vi "CC FITS Make FITS Header Table.vi"() -> ()   [LabVIEW 2021]
uses:
  typedefs/FITS HK Header Table.ctl
  Logging/CC enum Current Values Action.ctl
  <userlib>/gfitsio/cfitsio-bitpix.ctl
  <userlib>/gfitsio/gfitsio-write-image-subset-dbl-2d.vi
  hk-channel-class/HK Table/HK Table.lvclass
  <userlib>/gfitsio/gfitsio.lvlib
panel:
  in  "Fixed Header":bool
  in  "Test File":bool
  in  "Cancel Button":bool
  in  "OK Button":bool
  in  "Remove":bool
  in  "Add":bool
  in  "FITS Header":i32(listbox)
  in  "All Housekeeping":i32(listbox)
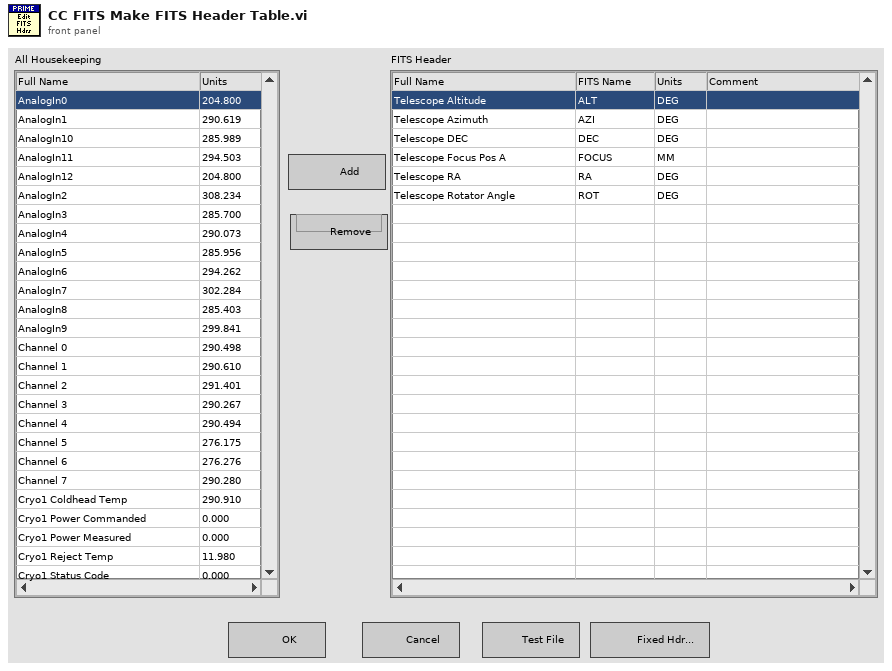
[diagram p1: front panel]
types:
  T1 = typedef "FITS HK Header Table.ctl" = cluster{"Full Name":string, "FITS Name":string, "Units":string, "Comment":string}
  T2 = cluster{"state":refnum<user-event>, "All HK":string[][], "Hdr Map":map{string, T1}, "Fixed Hdr":map{string, T1}}
  T3 = typedef "CC enum Current Values Action.ctl" = enum16{"Init", "Write Item", "Write Array", "Read Item", "Read Array", "Read All", "Add Channels", "New File", "Add Message", "Get Current Values", "Close"}
  T4 = enum16{"open", "open or create", "create", "create or replace"}
  T5 = enum16{"open", "open or create", "create or replace", "create", "open (read only)"}
  T6 = typedef "RIMAS Detector Config.ctl" = cluster{"Detector":u16, "Offsets":u16[][], "Detector Computer":T7, "FITS hdr template0":path, "FITS hdr template1":path, "FITS Data File Path":path, "FITS Detector Settings":T8, "Sim Folder":path, "Integration Mode":T9, "Integration Time":dbl, "Frame Int Time":dbl}
  T7 = typedef "RIMAS Detector Server Config.ctl" = cluster{"Machine":string, "Password":string, "FITS File Path":string, "Port":u16, "Header Path":string, "Name":string}
  T8 = typedef "RIMAS Observation Config.ctl" = cluster{"Exp Time Short":dbl, "# of Frames":dbl, "Exp Time Long":dbl, "# of Groups":dbl, "Object Name":string, "Object":string, "Obs Type":string, "Image Type":string, "Observer":string, "Observer Affiliation":string}
  T9 = typedef "Detector enum Detector Integration Mode.ctl" = enum16{"SSR", "CDS", "MEAN", "MEDIAN", "MODE", "MIIN", "MAX"}
  T10 = typedef "FITS cluster Header Row.ctl" = cluster{"Field Name":string, "Type":T11, "Value":string, "Comment":string, "Units":string}
  T11 = typedef "FITS enum Data Type.ctl" = enum16{"String", "Integer", "Float"}
  T12 = typedef "LVRowAndColumnTypeDef.ctl" = cluster{"Row":i32, "Column":i32}
  T13 = typedef "gfitsio.lvlib/cfitsio-bitpix.ctl" = i32
  T14 = typedef "gfitsio.lvlib/gfitsio-refnum.ctl" = refnum<k1>
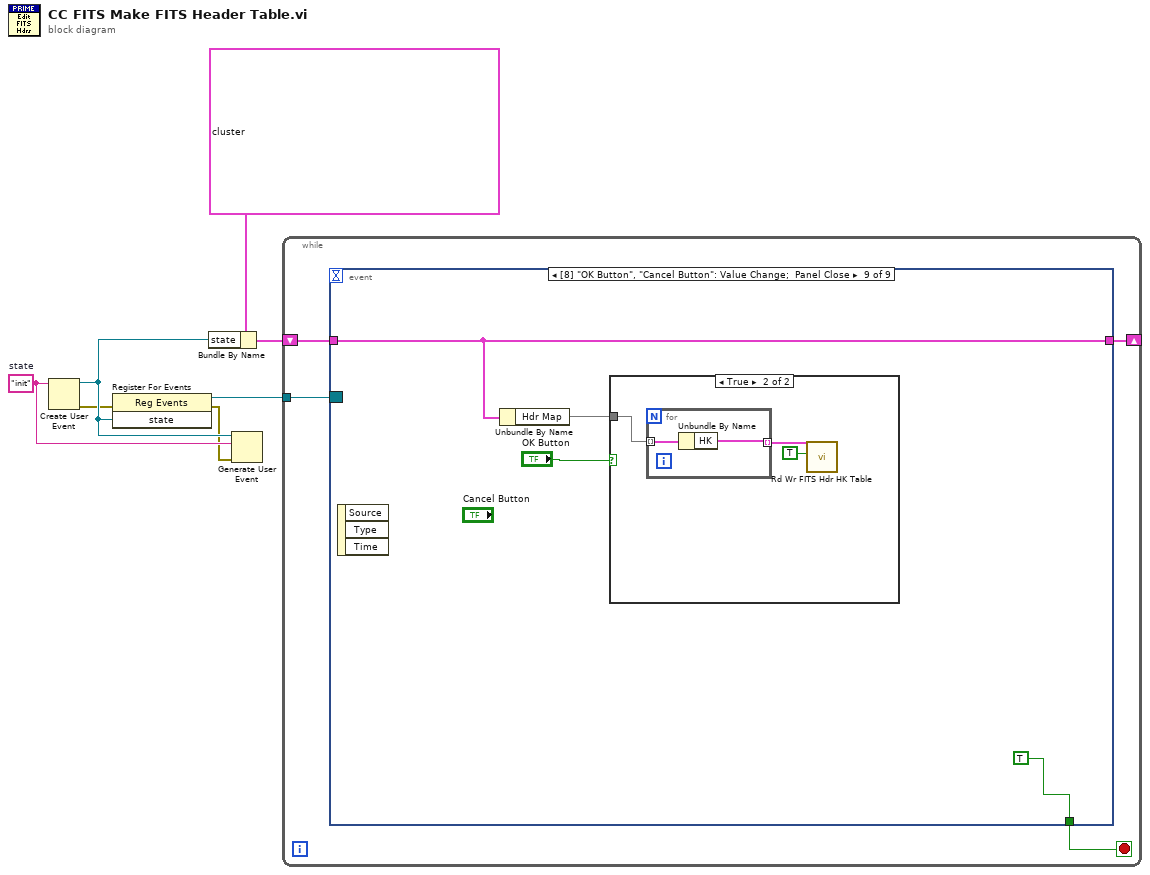
[diagram p0: block diagram]
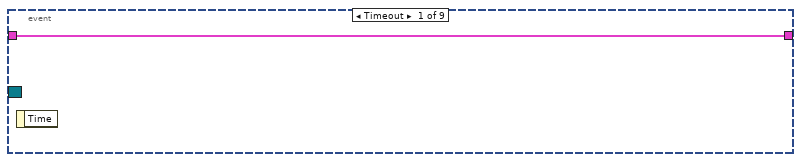
[diagram p2: hidden frame]
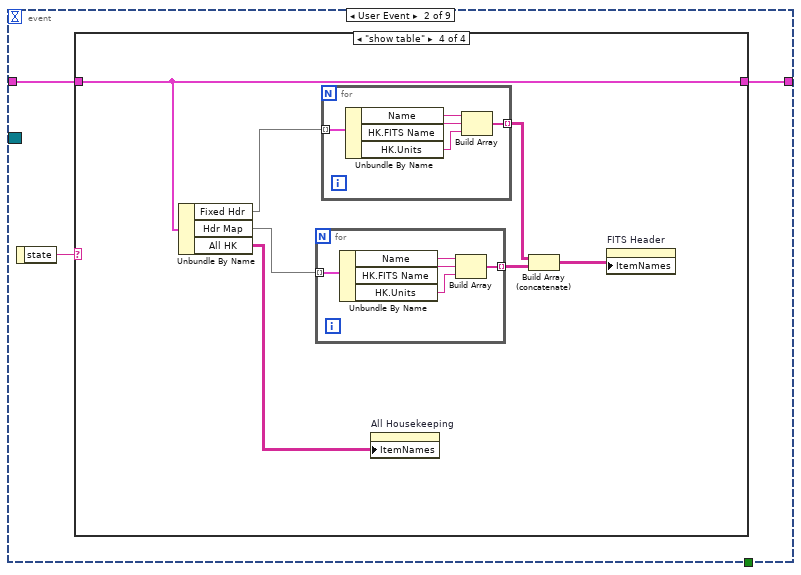
[diagram p3: hidden frame]
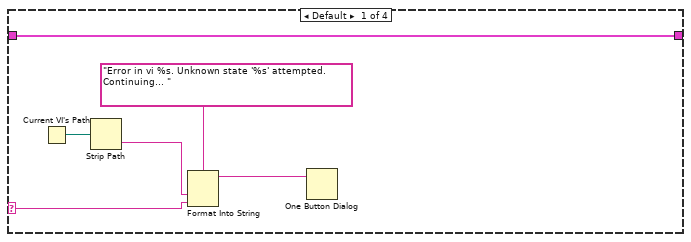
[diagram p4: hidden frame]
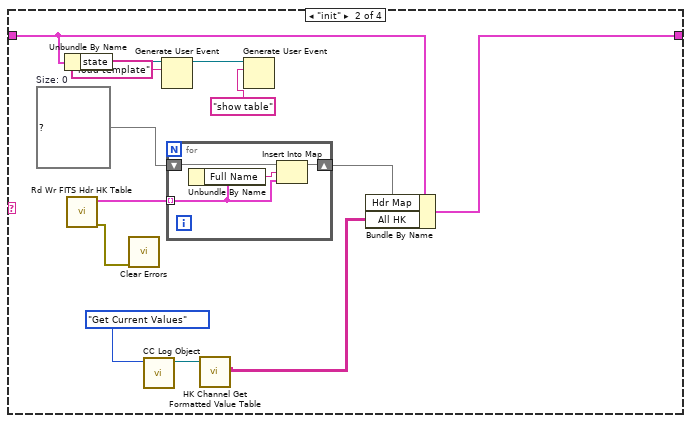
[diagram p5: hidden frame]
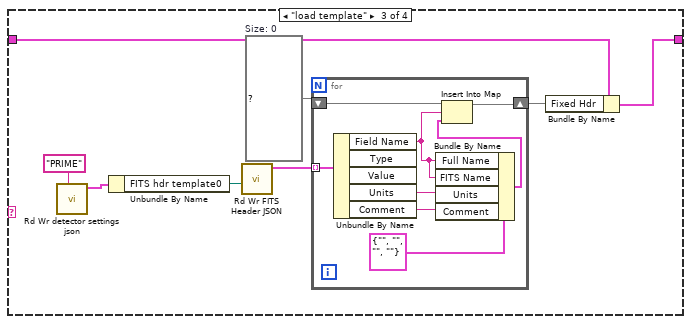
[diagram p6: hidden frame]
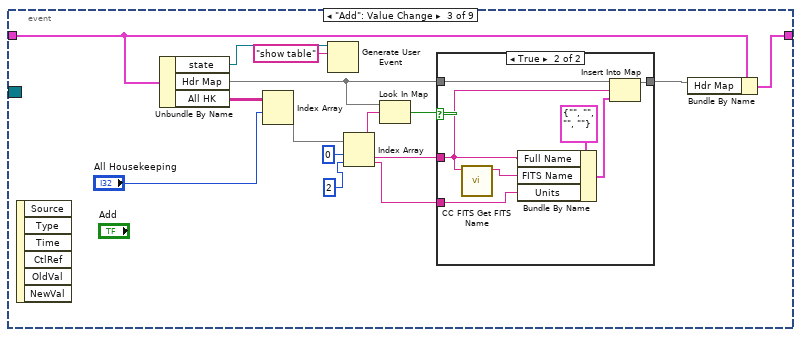
[diagram p7: hidden frame]
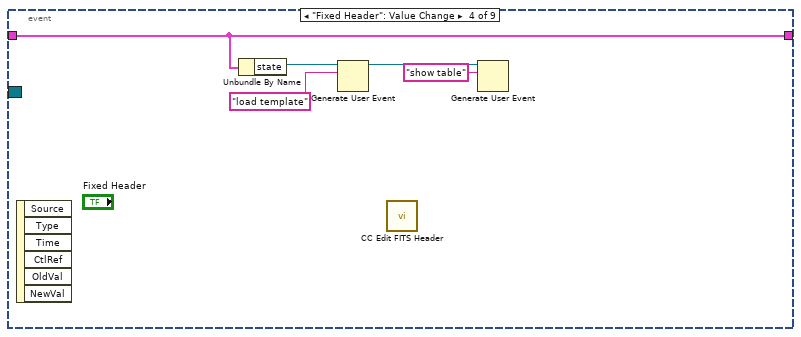
[diagram p9: hidden frame]
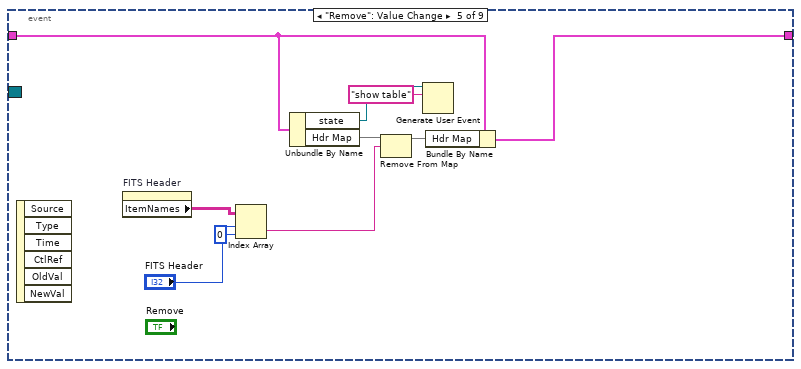
[diagram p10: hidden frame]
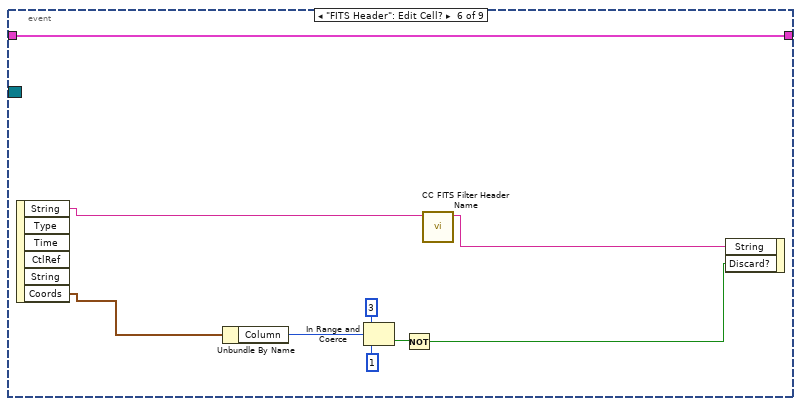
[diagram p11: hidden frame]
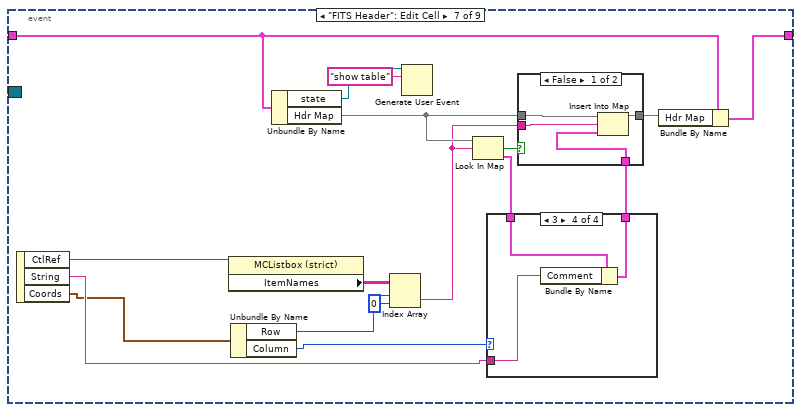
[diagram p12: hidden frame]
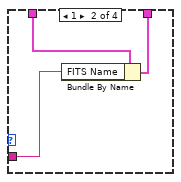
[diagram p14: hidden frame]
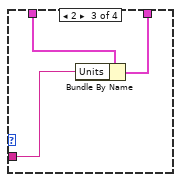
[diagram p15: hidden frame]
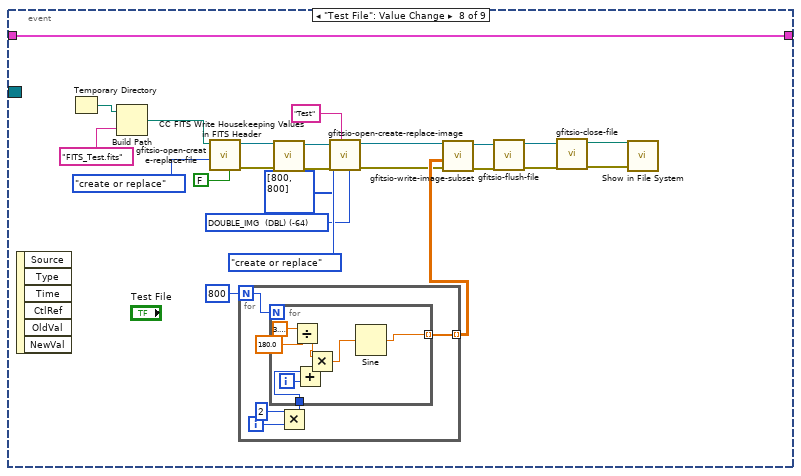
[diagram p17: hidden frame]
diagram:
  w3 = "init"  # state
  n1 = Create User Event(user event datatype=w3) -> (user event=w5:refnum<user-event>, error out=w1:errorcluster)  [unwired: 1 in]
  n2 = register-events(error in=w1, w5) -> (reference out=w4:refnum<event-registration>, error out=w2:errorcluster)  [unwired: 1 in]
  n3 = Bundle By Name(cluster=T2 {"state"=refnum, "All HK"=[], "Hdr Map"={}, "Fixed Hdr"={}}, "state"=w5) -> (w6:T2)
  n4 = Generate User Event(user event=w5, event data cluster=w3, error in=w2) -> ()  [unwired: 1 in, 2 out]
  n5 = while {
    tunnel: w4 -> [w11]
    shift-right: [w9] -> _
    shift-left: w6 -> [w10]
    stop <- w8 stop-if-true
    n6 = event shown="[8] \"OK Button\", \"Cancel Button\": Value Change;  Panel Close" {
      selector: w11 -> [_ _ _ _ _ _ _ _ _]
      dyn-events: _ -> [_ _ _ _ _ _ _ _ _]
      timeout: _ -> [_ _ _ _ _ _ _ _ _]
      tunnel: w10 -> [w12 w14 w74 w98 w101 w117 w128 w173 w188]
      tunnel: [w12 w13 w75 w98 w102 w117 w129 w173 w188] -> w9
      tunnel: [_ _ _ _ _ _ _ _ TRUE ("Close")] -> w8
      event Timeout {
        n7 = event-data() -> ()  [unwired: 1 in, 1 out]
      }
      event User Event {
        n8 = event-data() -> ("state"=w15:string)  [unwired: 1 in]
        n9 = case shown="\"show table\"" w15 {
          selector: w15 -> [w20 _ _ _]
          tunnel: w14 -> [w16 w31 w40 w61]
          tunnel: [w16 w32 w41 w61] -> w13
          frame Default {
            n10 = Current VI's Path() -> (path=w19:path)
            n11 = Strip Path(path=w19) -> (name=w18:string)  [unwired: 1 out]
            n12 = Format Into String(format string="Error in vi %s. Unknown state '%s' attempted. Continuing... ", w18, w20) -> (resulting string=w17:string)  [unwired: 2 in, 1 out]
            n13 = One Button Dialog(message=w17) -> ()  [unwired: 1 in, 1 out]
          }
          frame "init" {
            w27 = map{string, T1} {}  # Size: 0
            n14 = Unbundle By Name(w31) -> ("state"=w30:refnum<user-event>)
            n15 = call "Rd Wr FITS Hdr HK Table.vi"() -> ("error out"=w25:errorcluster, "FITS HK Hdr Table"=w28:T1[])  [unwired: 10 in]
            n16 = call <vilib>:"Clear Errors.vi"("error in (no error)"=w25) -> ()  [unwired: 5 in, 2 out]
            n17 = call "CC Log Object.vi"("Action"=CC_enum_Current_Values_Action."Get Current Values") -> ("HK Channel out"=w33:refnum<class "HK Table.lvclass">)  [unwired: 8 in, 2 out]
            n18 = Generate User Event(user event=w30, event data cluster="load template" ("event data")) -> (user event out=w23:refnum<user-event>)  [unwired: 2 in, 1 out]
            n19 = for {
              tunnel: w28 -> [w35] mode=indexing
              shift-right: [w36] -> w26
              shift-left: w27 -> [w37]
              n20 = Unbundle By Name(w35) -> ("Full Name"=w38:string)
              n21 = Insert Into Map(map in=w37, key=w38, value=w35) -> (map out=w36:map{string, T1})  [unwired: 2 out]
            }
            n22 = call-dynamic "HK Channel Get Formatted Value Table.vi"("HK Table in"=w33) -> ("Table"=w24:string[][])  [unwired: 6 in, 4 out]
            n23 = Generate User Event(user event=w23, event data cluster="show table" ("event data")) -> ()  [unwired: 2 in, 2 out]
            n24 = Bundle By Name(cluster=w31, "Hdr Map"=w26, "All HK"=w24) -> (w32:T2)
          }
          frame "load template" {
            w39 = map{string, T1} {}  # Size: 0
            n25 = call "Rd Wr detector settings json.vi"("Detector Name"="PRIME") -> ("Detector Config"=w45:T6)  [unwired: 9 in, 1 out]
            n26 = Unbundle By Name(w45) -> ("FITS hdr template0"=w44:path)
            n27 = call "Rd Wr FITS Header JSON.vi"("FITS Template"=w44) -> ("FITS Hdr Rows"=w43:T10[])  [unwired: 9 in, 1 out]
            n28 = for {
              tunnel: w43 -> [w54] mode=indexing
              shift-right: [w47] -> w42
              shift-left: w39 -> [w53]
              n29 = Unbundle By Name(w54) -> ("Field Name"=w51:string, "Units"=w50:string, "Comment"=w49:string)  [unwired: 2 out]
              n30 = Bundle By Name(cluster=T1 {"Full Name"="", "FITS Name"="", "Units"="", "Comment"=""} ("value"), "Full Name"=w51, "FITS Name"=w51, "Units"=w50, "Comment"=w49) -> (w48:T1)
              n31 = Insert Into Map(map in=w53, key=w51, value=w48) -> (map out=w47:map{string, T1})  [unwired: 2 out]
            }
            n32 = Bundle By Name(cluster=w40, "Fixed Hdr"=w42) -> (w41:T2)
          }
          frame "show table" {
            n33 = Unbundle By Name(w61) -> ("Fixed Hdr"=w57:map{string, T1}, "Hdr Map"=w60:map{string, T1}, "All HK"=w58:string[][])
            n34 = for {
              tunnel: w60 -> [w71] mode=indexing
              tunnel: [w67] -> w59 mode=indexing
              n35 = Unbundle By Name(w71) -> ("Name"=w70:string, "HK.FITS Name"=w69:string, "HK.Units"=w68:string)
              n36 = Build Array(w70, w69, w68) -> (w67:string[])
            }
            n37 = for {
              tunnel: w57 -> [w66] mode=indexing
              tunnel: [w62] -> w55 mode=indexing
              n38 = Unbundle By Name(w66) -> ("Name"=w65:string, "HK.FITS Name"=w64:string, "HK.Units"=w63:string)
              n39 = Build Array(w65, w64, w63) -> (w62:string[])
            }
            n40 = property on="All Housekeeping" class="MCListbox (strict)"("ItemNames"=w58) -> ()  [unwired: 2 in, 2 out]
            n41 = Build Array (concatenate)(w55, w59) -> (w56:string[][])
            n42 = property on="FITS Header" class="MCListbox (strict)"("ItemNames"=w56) -> ()  [unwired: 2 in, 2 out]
          }
        }
      }
      event "Add": Value Change {
        n43 = event-data() -> ()  [unwired: 1 in, 6 out]
        n44 = Unbundle By Name(w74) -> ("state"=w73:refnum<user-event>, "Hdr Map"=w78:map{string, T1}, "All HK"=w85:string[][])
        n45 = Index Array(array=w85, index (row)="All Housekeeping") -> (element=w83:string[])  [unwired: 1 in]
        n46 = Generate User Event(user event=w73, event data cluster="show table" ("event data")) -> ()  [unwired: 2 in, 2 out]
        n47 = Index Array(array=w83, index #1=0 ("index"), index #2=2 ("index")) -> (element #1=w79:string, element #2=w77:string)
        n48 = Look In Map(map=w78, key=w79) -> (key not found?=w80:bool)  [unwired: 1 in, 1 out]
        n49 = case shown="True" w80 {
          tunnel: w79 -> [_ w90]
          tunnel: w78 -> [w86 w93]
          tunnel: w77 -> [_ w88]
          tunnel: [w86 w87] -> w76
          frame False {
          }
          frame True {
            n50 = call "CC FITS Get FITS Name.vi"("Full Name"=w90) -> ("FITS Hdr Name"=w91:string)  [unwired: 9 in, 1 out]
            n51 = Bundle By Name(cluster=T1 {"Full Name"="", "FITS Name"="", "Units"="", "Comment"=""} ("value"), "Full Name"=w90, "FITS Name"=w91, "Units"=w88) -> (w89:T1)
            n52 = Insert Into Map(map in=w93, key=w90, value=w89) -> (map out=w87:map{string, T1})  [unwired: 2 out]
          }
        }
        n53 = Bundle By Name(cluster=w74, "Hdr Map"=w76) -> (w75:T2)
      }
      event "Fixed Header": Value Change {
        n54 = event-data() -> ()  [unwired: 1 in, 6 out]
        n55 = Unbundle By Name(w98) -> ("state"=w97:refnum<user-event>)
        n56 = Generate User Event(user event=w97, event data cluster="load template" ("event data")) -> (user event out=w95:refnum<user-event>)  [unwired: 2 in, 1 out]
        n57 = call "CC Edit FITS Header.vi"() -> ()  [unwired: 12 in]
        n58 = Generate User Event(user event=w95, event data cluster="show table" ("event data")) -> ()  [unwired: 2 in, 2 out]
      }
      event "Remove": Value Change {
        n59 = event-data() -> ()  [unwired: 1 in, 6 out]
        n60 = property on="FITS Header" class="MCListbox (strict)"() -> ("ItemNames"=w108:string[][])  [unwired: 2 in, 2 out]
        n61 = Index Array(array=w108, index (row)="FITS Header", index (col)=0 ("disabled index (col)")) -> (element=w104:string)
        n62 = Unbundle By Name(w101) -> ("state"=w100:refnum<user-event>, "Hdr Map"=w105:map{string, T1})
        n63 = Remove From Map(10:w104, 11:w105) -> (3:w103:map{string, T1})  [unwired: 2 out]
        n64 = Generate User Event(user event=w100, event data cluster="show table" ("event data")) -> ()  [unwired: 2 in, 2 out]
        n65 = Bundle By Name(cluster=w101, "Hdr Map"=w103) -> (w102:T2)
      }
      event "FITS Header": Edit Cell? {
        n66 = event-data() -> ("String"=w112:string, "Coords"=w110:T12)  [unwired: 1 in, 4 out]
        n67 = Unbundle By Name(w110) -> ("Column"=w113:i32)
        n68 = In Range and Coerce(upper limit=3, x=w113, lower limit=1) -> (In Range?=w114:bool)  [unwired: 1 out]
        n69 = Not(x=w114) -> (.not. x?=w109:bool)
        n70 = call "CC FITS Filter Header Name.vi"("FITS Name In"=w112) -> ("FITS Name Out"=w111:string)  [unwired: 9 in, 1 out]
        n71 = event-data("String"=w111, "Discard?"=w109) -> ()  [unwired: 1 in, 1 out]
      }
      event "FITS Header": Edit Cell {
        n72 = event-data() -> ("CtlRef"=w118:refnum<vi>, "String"=w122:string, "Coords"=w119:T12)  [unwired: 1 in]
        n73 = property class="MCListbox (strict)"(reference=w118) -> ("ItemNames"=w134:string[][])  [unwired: 1 in, 2 out]
        n74 = Unbundle By Name(w119) -> ("Row"=w133:i32, "Column"=w123:i32)
        n75 = Unbundle By Name(w128) -> ("state"=w127:refnum<user-event>, "Hdr Map"=w132:map{string, T1})
        n76 = Index Array(array=w134, index (row)=w133, index (col)=0 ("disabled index (col)")) -> (element=w120:string)
        n77 = Generate User Event(user event=w127, event data cluster="show table" ("event data")) -> ()  [unwired: 2 in, 2 out]
        n78 = Look In Map(map=w132, key=w120) -> (key not found?=w131:bool, value=w125:T1)  [unwired: 1 in]
        n79 = case shown="3" w123 {
          tunnel: w125 -> [w135 w138 w141 w144]
          tunnel: [w135 w137 w140 w143] -> w124
          tunnel: w122 -> [_ w136 w139 w142]
          frame 0, Default {
          }
          frame 1 {
            n80 = Bundle By Name(cluster=w138, "FITS Name"=w136) -> (w137:T1)
          }
          frame 2 {
            n81 = Bundle By Name(cluster=w141, "Units"=w139) -> (w140:T1)
          }
          frame 3 {
            n82 = Bundle By Name(cluster=w144, "Comment"=w142) -> (w143:T1)
          }
        }
        n83 = case shown="False" w131 {
          tunnel: w132 -> [w148 w149]
          tunnel: w120 -> [w147 _]
          tunnel: [w146 w149] -> w130
          tunnel: w124 -> [w145 _]
          frame False {
            n84 = Insert Into Map(map in=w148, key=w147, value=w145) -> (map out=w146:map{string, T1})  [unwired: 2 out]
          }
          frame True {
          }
        }
        n85 = Bundle By Name(cluster=w128, "Hdr Map"=w130) -> (w129:T2)
      }
      event "Test File": Value Change {
        w150 = T13 -64 items=["<invalid type>"=0, "BYTE_IMG  (U8)"=8, "SHORT_IMG  (I16)"=16, "USHORT_IMG  (U16)"=20, "LONG_IMG  (I32)"=32, "ULONG_IMG  (U32)"=40, "FLOAT_IMG  (SGL)"=-32, "DOUBLE_IMG  (DBL)"=-64] ("image data type")
        n86 = event-data() -> ()  [unwired: 1 in, 6 out]
        n87 = Temporary Directory() -> (w170:path)
        n88 = Build Path(base path=w170, name or relative path="FITS_Test.fits") -> (appended path=w168:path)
        n89 = call <userlib>:"gfitsio-open-create-replace-file.vi"("advisory dialog? (display:T)"=FALSE, "function (open)"=T5."create or replace", "file path (dialog if empty)"=w168) -> ("error out"=w172:errorcluster, "gfits refnum"=w171:T14)  [unwired: 6 in, 1 out]
        n90 = for {
          N: 800 -> [w178]
          tunnel: [w175] -> w164 mode=indexing
          i -> [w177]
          n91 = Multiply(x=2, y=w177) -> (x*y=w174:i32)
          n92 = for {
            N: w178 -> [_]
            tunnel: [w181] -> w175 mode=indexing
            tunnel: w174 -> [w179]
            i -> [w186]
            n93 = Divide(x=3.141592653589793, y=180.0) -> (x/y=w183:dbl)
            n94 = Add(x=w179, y=w186) -> (x+y=w180:i32)
            n95 = Multiply(x=w183, y=w180) -> (x*y=w182:dbl)
            n96 = Sine(x=w182) -> (sin(x)=w181:dbl)
          }
        }
        n97 = call "CC FITS Write Housekeeping Values in FITS Header.vi"("error in (no error)"=w172, "gfits refnum"=w171) -> ("error out"=w157:errorcluster, "dup gfits refnum"=w156:T14)  [unwired: 8 in]
        n98 = call <userlib>:"gfitsio-open-create-replace-image.vi"("image data type"=w150, "hdu name (dialog if empty)"="Test", "error in (no error)"=w157, "function (create or replace)"=T4."create or replace", "naxes"=i32[] [800, 800], "gfits refnum"=w156) -> ("error out"=w151:errorcluster, "dup gfits refnum"=w152:T14)  [unwired: 3 in, 1 out]
        n99 = call-poly <userlib>:"gfitsio-write-image-subset.vi"("error in (no error)"=w151, "data"=w164, "gfits refnum"=w152) -> ("error out"=w163:errorcluster, "dup gfits refnum"=w162:T14)  [unwired: 7 in]
        n100 = call <userlib>:"gfitsio-flush-file.vi"("error in (no error)"=w163, "gfits refnum"=w162) -> ("error out"=w160:errorcluster, "dup gfits refnum"=w161:T14)  [unwired: 8 in]
        n101 = call <userlib>:"gfitsio-close-file.vi"("error in (no error)"=w160, "gfits refnum"=w161) -> ("error out"=w158:errorcluster, "Path"=w159:path)  [unwired: 8 in]
        n102 = call <vilib>:"Show in File System.vi"("error in (no error)"=w158, "file or directory path"=w159) -> ()  [unwired: 9 in, 1 out]
      }
      event "OK Button", "Cancel Button": Value Change; Panel Close {
        n103 = event-data() -> ()  [unwired: 1 in, 3 out]
        n104 = Unbundle By Name(w188) -> ("Hdr Map"=w187:map{string, T1})
        n105 = case shown="True" "OK Button" {
          tunnel: w187 -> [_ w193]
          frame False {
          }
          frame True {
            n106 = for {
              tunnel: w193 -> [w195] mode=indexing
              tunnel: [w194] -> w192 mode=indexing
              n107 = Unbundle By Name(w195) -> ("HK"=w194:T1)
            }
            n108 = call "Rd Wr FITS Hdr HK Table.vi"("Write? (F:Read)"=TRUE, "FITS HK Hdr Table"=w192) -> ()  [unwired: 8 in, 2 out]
          }
        }
      }
    }
  }
